vi "Max_forsed_bit32.vi"(3 "IN":u32 format="%b") -> (1 "N":u32 format="%b")   [LabVIEW 2015]
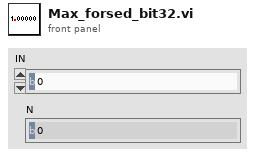
[diagram p1: front panel]
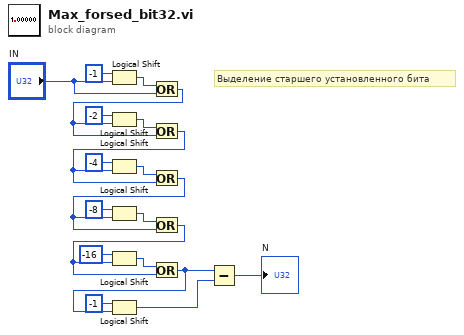
[diagram p0: block diagram]
diagram:
  # "Выделение старшего установленного бита"
  n1 = Logical Shift(y=i16 -1, x="IN") -> (x << y=w11:u32)
  n2 = Or(x=w11, y="IN") -> (x .or. y?=w10:u32)
  n3 = Logical Shift(y=i16 -2, x=w10) -> (x << y=w18:u32)
  n4 = Or(x=w18, y=w10) -> (x .or. y?=w9:u32)
  n5 = Logical Shift(y=i16 -4, x=w9) -> (x << y=w15:u32)
  n6 = Or(x=w15, y=w9) -> (x .or. y?=w8:u32)
  n7 = Logical Shift(y=i16 -8, x=w8) -> (x << y=w14:u32)
  n8 = Or(x=w14, y=w8) -> (x .or. y?=w3:u32)
  n9 = Logical Shift(y=i16 -16, x=w3) -> (x << y=w4:u32)
  n10 = Or(x=w4, y=w3) -> (x .or. y?=w1:u32)
  n11 = Logical Shift(y=i16 -1, x=w1) -> (x << y=w7:u32)
  n12 = Subtract(x=w1, y=w7) -> (x-y=→"N":u32)
